vi "Get Start and Stop VS Channel Handles for Terminals.vi"(8 "error in":errorcluster, 11 "custom device ref":T1 format="%.0x") -> (0 "error out":errorcluster, 2 "start stop channel handles":T1[](array[typedef]) format="%.0x", 3 "running status channel handles":T1[](array[typedef]) format="%.0x")   [LabVIEW 2020, in "AIM MIL-STD-1553 Engine.lvlib" / "Implementation.lvlib" / "Triggers Execution Unit.lvclass"]
uses:
  Triggers Execution Unit.lvclass
  <vilib>/NI VeriStand/Custom Device API/Custom Device Item Ref.ctl
  Scripting/AIM MIL-STD-1553 Scripting.lvlib
  <vilib>/NI VeriStand/Custom Device API/Custom Device API.lvlib
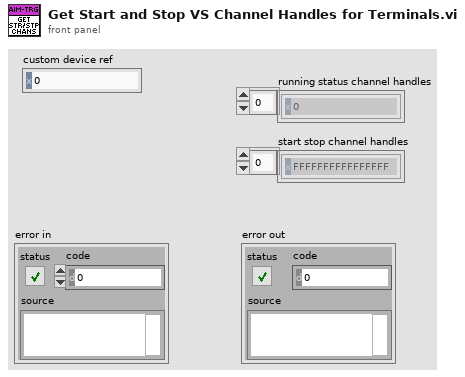
[diagram p1: front panel]
types:
  T1 = typedef "Custom Device API.lvlib/Custom Device Item Ref.ctl" = u64
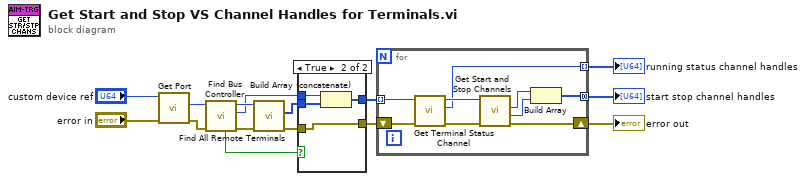
[diagram p0: block diagram]
diagram:
  n1 = call "Get Port.vi"("error in"="error in", "custom device ref"="custom device ref") -> ("error out"=w12:errorcluster, "port"=w13:T1)  [unwired: 6 in, 2 out]
  n2 = call "Find Bus Controller.vi"("error in"=w12, "port"=w13) -> ("error out"=w10:errorcluster, "bus controller"=w6:T1, "port out"=w11:T1, "found?"=w3:bool)  [unwired: 6 in]
  n3 = call "Find All Remote Terminals.vi"("error in"=w10, "port"=w11) -> ("error out"=w1:errorcluster, "remote terminals"=w5:T1[])  [unwired: 7 in, 1 out]
  n4 = case shown="True" w3 {
    tunnel: [w17 w21] -> w7
    tunnel: w6 -> [_ w20]
    tunnel: w5 -> [w17 w19]
    tunnel: [w16 w18] -> w2
    tunnel: w1 -> [w16 w18]
    frame False {
    }
    frame True {
      n5 = Build Array (concatenate)(w20, w19) -> (w21:T1[])
    }
  }
  n6 = for {
    shift-right: [w30] -> w9
    shift-left: w2 -> [w26]
    tunnel: [w27] -> w8 mode=concatenating
    tunnel: w7 -> [w24] mode=indexing
    tunnel: [w22] -> w4 mode=indexing
    n7 = call "Get Terminal Status Channel.vi"("error in"=w26, "terminal"=w24) -> ("error out"=w25:errorcluster, "status channel"=w22:T1, "terminal out"=w23:T1)  [unwired: 6 in, 1 out]
    n8 = call "Get Start and Stop Channels.vi"("error in"=w25, "terminal"=w23) -> ("error out"=w30:errorcluster, "stop channel"=w28:T1, "start channel"=w29:T1)  [unwired: 5 in, 2 out]
    n9 = Build Array(w29, w28) -> (w27:T1[])
  }
  "error out" <- w9
  "start stop channel handles" <- w8
  "running status channel handles" <- w4
